vi "Replace with Property Values.vi"(9 "SLSC Switch States in":T1, 10 "replace string":string="SLSC-12001-0317E1AA-Mod2", 11 "search string":string="SLSC 1225x Module 1") -> (1 "SLSC Switch States out":T1)   [LabVIEW 2017, in "SLSC Switch System Tests.lvclass"]
uses:
  SLSC Switch System Tests.lvclass
  SLSC Switch States.ctl
panel:
  # "SLSC-12001-0317E1AA-Mod2"
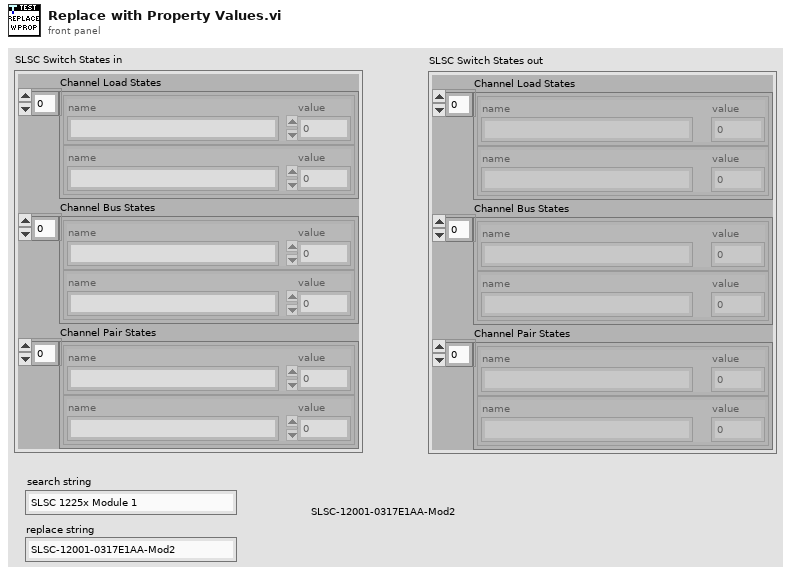
[diagram p1: front panel]
types:
  T1 = typedef "SLSC Switch System Tests.lvclass/SLSC Switch States.ctl" = cluster{"Channel Load States":cluster{"name":string, "value":i32}[], "Channel Bus States":cluster{"name":string, "value":i32}[], "Channel Pair States":cluster{"name":string, "value":i32}[]}
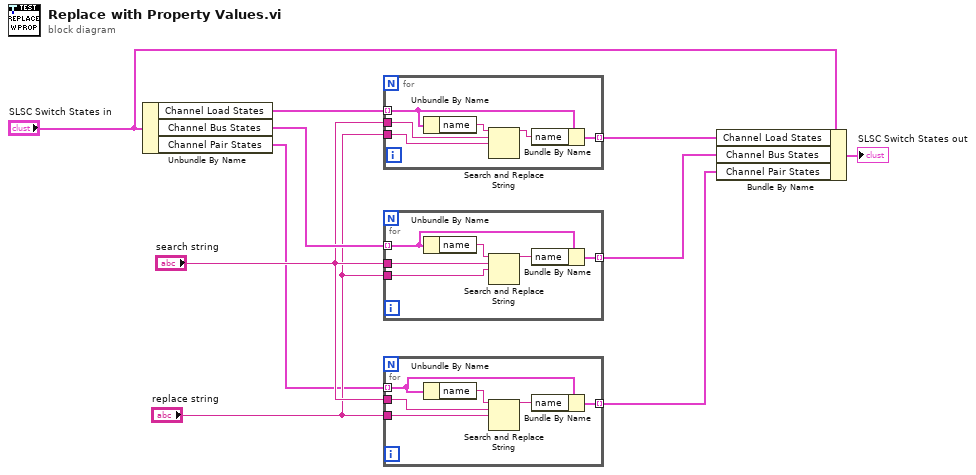
[diagram p0: block diagram]
diagram:
  n1 = Unbundle By Name("SLSC Switch States in") -> ("Channel Load States"=w10:cluster{"name":string, "value":i32}[], "Channel Bus States"=w6:cluster{"name":string, "value":i32}[], "Channel Pair States"=w2:cluster{"name":string, "value":i32}[])
  n2 = for {
    tunnel: w10 -> [w13] mode=indexing
    tunnel: "search string" -> [w15]
    tunnel: "replace string" -> [w14]
    tunnel: [w11] -> w8 mode=indexing
    n3 = Unbundle By Name(w13) -> ("name"=w16:string)
    n4 = Search and Replace String(input string=w16, search string=w15, replace string=w14) -> (result string=w12:string)  [unwired: 5 in, 3 out]
    n5 = Bundle By Name(cluster=w13, "name"=w12) -> (w11:cluster{"name":string, "value":i32})
  }
  n6 = for {
    tunnel: w6 -> [w19] mode=indexing
    tunnel: "search string" -> [w21]
    tunnel: "replace string" -> [w20]
    tunnel: [w17] -> w1 mode=indexing
    n7 = Unbundle By Name(w19) -> ("name"=w22:string)
    n8 = Search and Replace String(input string=w22, search string=w21, replace string=w20) -> (result string=w18:string)  [unwired: 5 in, 3 out]
    n9 = Bundle By Name(cluster=w19, "name"=w18) -> (w17:cluster{"name":string, "value":i32})
  }
  n10 = for {
    tunnel: w2 -> [w25] mode=indexing
    tunnel: "search string" -> [w27]
    tunnel: "replace string" -> [w26]
    tunnel: [w23] -> w3 mode=indexing
    n11 = Unbundle By Name(w25) -> ("name"=w28:string)
    n12 = Search and Replace String(input string=w28, search string=w27, replace string=w26) -> (result string=w24:string)  [unwired: 5 in, 3 out]
    n13 = Bundle By Name(cluster=w25, "name"=w24) -> (w23:cluster{"name":string, "value":i32})
  }
  n14 = Bundle By Name(cluster="SLSC Switch States in", "Channel Load States"=w8, "Channel Bus States"=w1, "Channel Pair States"=w3) -> (→"SLSC Switch States out":T1)
